vi "getdllversion.vi"(8 "error in (no error)":errorcluster) -> (0 "error out":errorcluster, 2 "DLLVersion":i32 format="%.0x")   [LabVIEW 2009]
doc: "This VI returns the neoVI DLL Version.\n\n12/21/2010 1.0.0 jyg\n- initial release"
uses:
  NEO VI Example/data/icsneo40.dll
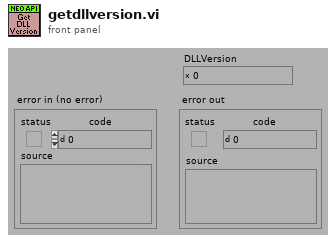
[diagram p1: front panel]
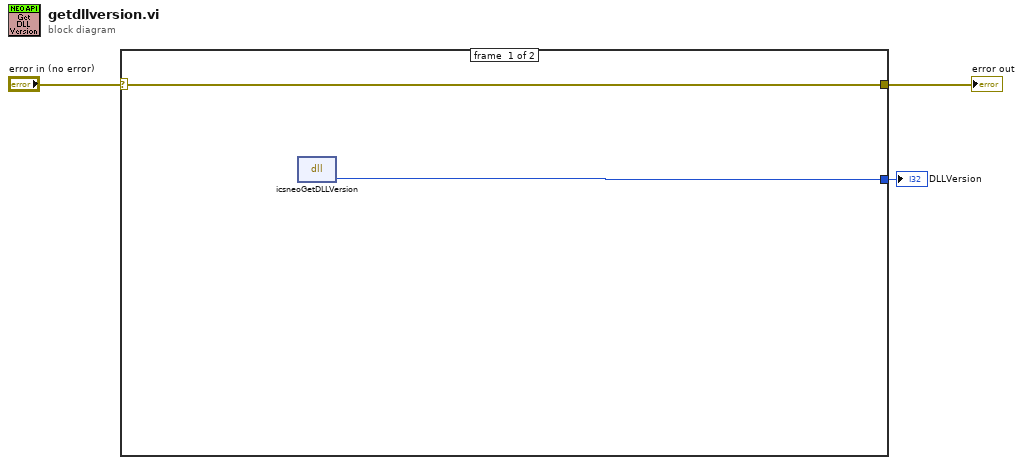
[diagram p0: block diagram]
diagram:
  n1 = case shown="No Error" "error in (no error)" {
    selector: "error in (no error)" -> [w5 w6]
    tunnel: [w5 w6] -> w3
    tunnel: [w4 _] -> w1
    frame #0 {
      n2 = dll-call lib="C:/WINDOWS/system32/icsneo40.dll" fn="icsneoGetDLLVersion"() -> ("return type"=w4:i32)  [unwired: 3 in, 2 out]
    }
    frame #1 {
    }
  }
  "error out" <- w3
  "DLLVersion" <- w1
